vi "Create Test Library from Template.vi"() -> ()   [LabVIEW 2016]
doc: "This VI creates and adds the Drona test library template to the active project"
panel:
  out "error out":errorcluster
  in  "error in (no error)":errorcluster
  in  "Library Name":string="TestLibrary.lvlib"
  # "Creating Drona Test Library\nfrom Template......"
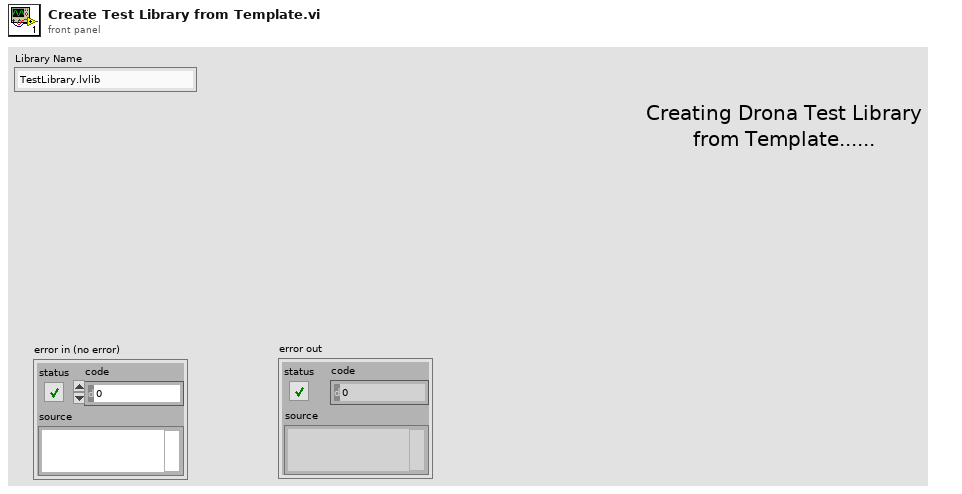
[diagram p1: front panel]
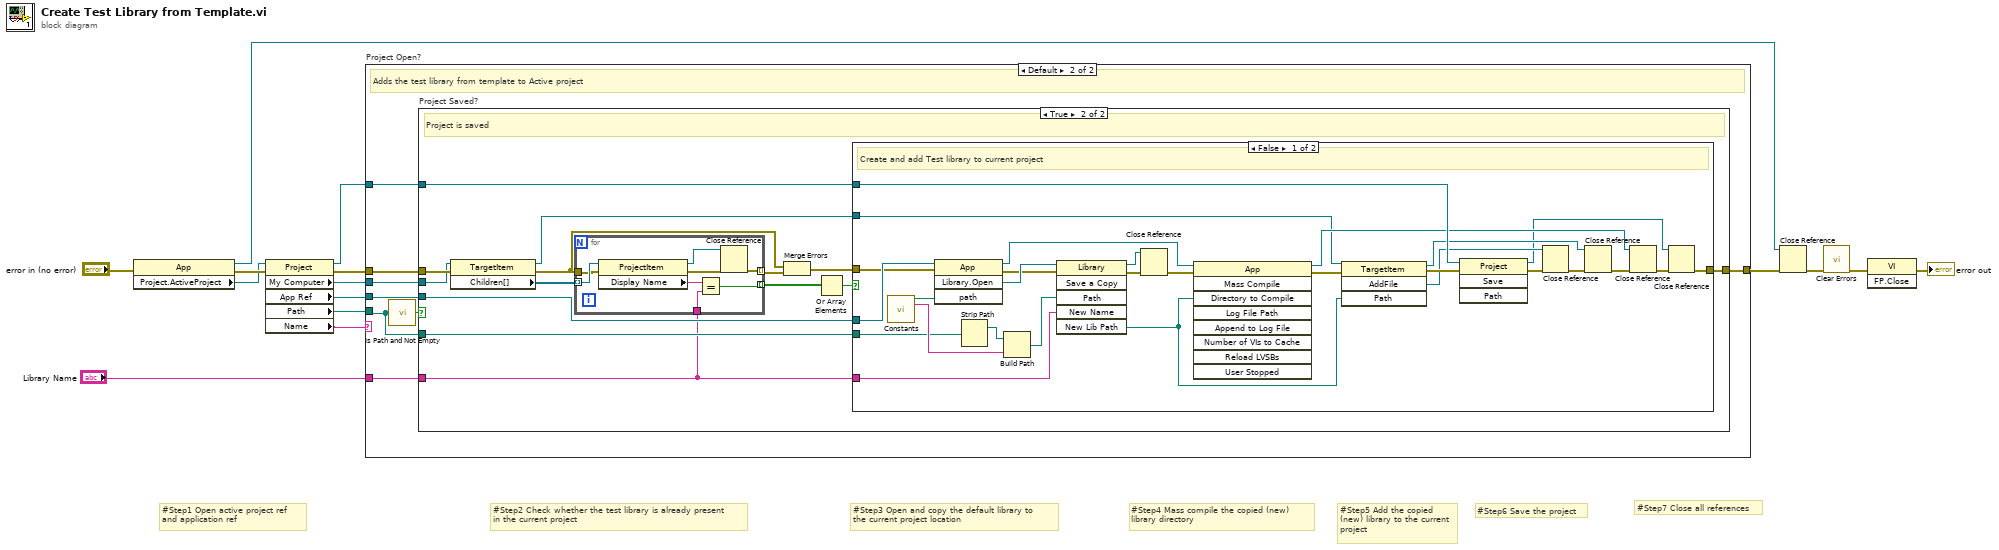
[diagram p0: block diagram]
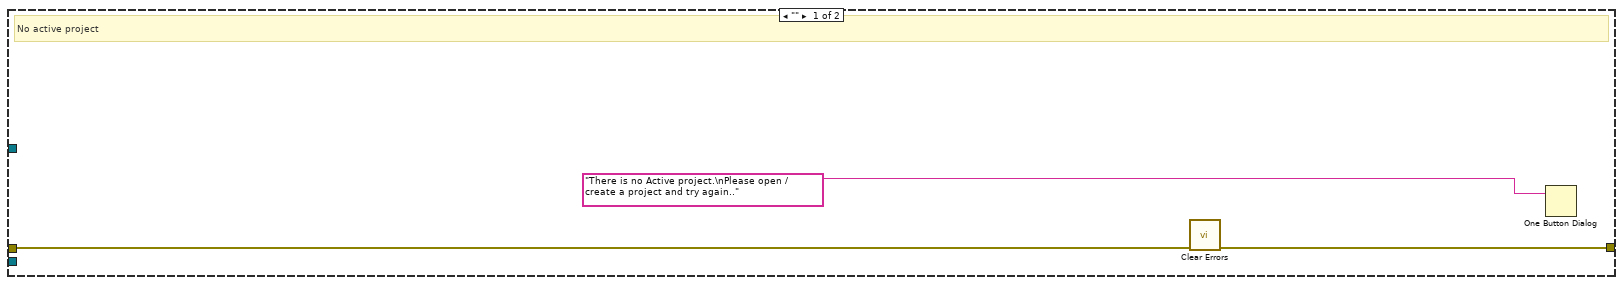
[diagram p2: hidden frame]
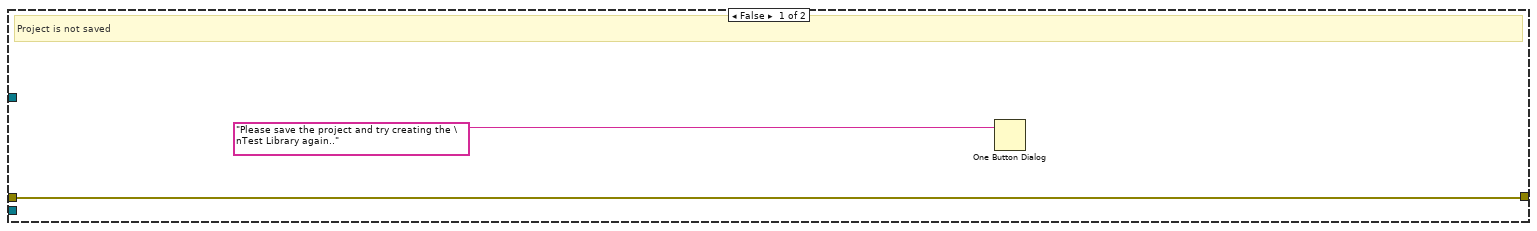
[diagram p3: hidden frame]
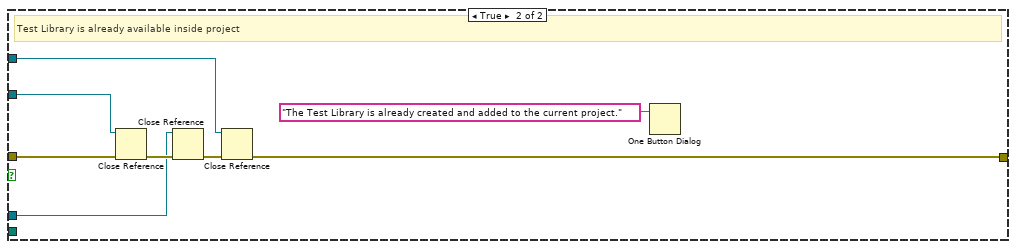
[diagram p4: hidden frame]
diagram:
  # "#Step7 Close all references"
  # "#Step6 Save the project"
  # "#Step5 Add the copied (new) library to the current project"
  # "#Step4 Mass compile the copied (new) \nlibrary directory"
  # "#Step3 Open and copy the default library to \nthe current project location"
  # "#Step2 Check whether the test library is already present\nin the current project"
  # "#Step1 Open active project ref \nand application ref"
  n1 = property class="App"(error in="error in (no error)") -> (reference out=w12:refnum<vi>, error out=w15:errorcluster, "Project.ActiveProject"=w11:refnum<vi>)  [unwired: 1 in]
  n2 = property class="Project"(reference=w11, error in=w15) -> (reference out=w2:refnum<vi>, error out=w14:errorcluster, "My Computer"=w3:refnum<vi>, "App Ref"=w13:refnum<vi>, "Path"=w10:path, "Name"=w9:string)
  n3 = case "Project Open?" shown="Default" w9 {
    tunnel: w3 -> [_ w21]
    tunnel: w14 -> [w18 w24]
    tunnel: w13 -> [_ w25]
    tunnel: [w17 w19] -> w1
    tunnel: w10 -> [_ w23]
    tunnel: "Library Name" -> [_ w22]
    tunnel: w2 -> [_ w20]
    frame "" {
      # "No active project"
      n4 = call <vilib>:"Clear Errors.vi"("error in (no error)"=w18) -> ("error out"=w17:errorcluster)  [unwired: 5 in, 1 out]
      n5 = One Button Dialog(message="There is no Active project.\nPlease open / create a project and try again..") -> ()  [unwired: 1 in, 1 out]
    }
    frame Default {
      # "Adds the test library from template to Active project"
      n6 = call <vilib>:"Is Path and Not Empty.vi"("path"=w23) -> ("Is Path and Not Empty?"=w26:bool)  [unwired: 4 in]
      n7 = case "Project Saved?" shown="True" w26 {
        tunnel: w25 -> [_ w42]
        tunnel: w24 -> [w28 w38]
        tunnel: w23 -> [_ w41]
        tunnel: w22 -> [_ w34]
        tunnel: w21 -> [_ w37]
        tunnel: w20 -> [_ w40]
        tunnel: [w28 w39] -> w19
        frame False {
          # "Project is not saved"
          n8 = One Button Dialog(message="Please save the project and try creating the \nTest Library again..") -> ()  [unwired: 1 in, 1 out]
        }
        frame True {
          # "Project is saved"
          n9 = property class="TargetItem"(reference=w37, error in=w38) -> (reference out=w36:refnum<vi>, error out=w31:errorcluster, "Children[]"=w35:refnum<vi>[])
          n10 = for {
            tunnel: w35 -> [w86] mode=indexing
            tunnel: w31 -> [w85]
            tunnel: w34 -> [w83]
            tunnel: [w82] -> w33 mode=indexing
            tunnel: [w79] -> w32 mode=indexing
            n11 = property class="ProjectItem"(reference=w86, error in=w85) -> (reference out=w81:refnum<vi>, error out=w80:errorcluster, "Display Name"=w84:string)
            n12 = Equal?(x=w84, y=w83) -> (x = y?=w82:bool)
            n13 = Close Reference(reference=w81, error in (no error)=w80) -> (error out=w79:errorcluster)
          }
          n14 = Merge Errors(w31, w32) -> (w30:errorcluster)
          n15 = Or Array Elements(Boolean array=w33) -> (logical OR=w29:bool)
          n16 = case shown="False" w29 {
            tunnel: w42 -> [w70 w76]
            tunnel: w41 -> [w64 _]
            tunnel: w40 -> [w55 w74]
            tunnel: [w46 w72] -> w39
            tunnel: w36 -> [w45 w78]
            tunnel: w34 -> [w44 _]
            tunnel: w30 -> [w43 w73]
            frame False {
              # "Create and add Test library to current project"
              n17 = call "Constants.vi"() -> ("VI path"=w69:path, "Tests folder name"=w65:string)  [unwired: 14 in]
              n18 = invoke class="App" method="Library.Open"(reference=w70, error in=w43, "path"=w69) -> (reference out=w60:refnum<vi>, error out=w67:errorcluster, "Open Library"=w68:refnum<vi>)  [unwired: 1 in, 1 out]
              n19 = Strip Path(path=w64) -> (stripped path=w66:path)  [unwired: 1 out]
              n20 = Build Path(base path=w66, name or relative path=w65) -> (appended path=w63:path)
              n21 = invoke class="Library" method="Save a Copy"(reference=w68, error in=w67, "Path"=w63, "New Name"=w44) -> (reference out=w61:refnum<vi>, error out=w62:errorcluster, "New Lib Path"=w57:path)  [unwired: 2 in, 3 out]
              n22 = Close Reference(reference=w61, error in (no error)=w62) -> (error out=w59:errorcluster)
              n23 = invoke class="App" method="Mass Compile"(reference=w60, error in=w59, "Directory to Compile"=w57) -> (reference out=w49:refnum<vi>, error out=w58:errorcluster)  [unwired: 6 in, 7 out]
              n24 = invoke class="TargetItem" method="AddFile"(reference=w45, error in=w58, "Path"=w57) -> (reference out=w51:refnum<vi>, error out=w56:errorcluster, "AddFile"=w52:refnum<vi>)  [unwired: 1 in, 1 out]
              n25 = invoke class="Project" method="Save"(reference=w55, error in=w56) -> (reference out=w47:refnum<vi>, error out=w54:errorcluster)  [unwired: 2 in, 2 out]
              n26 = Close Reference(reference=w52, error in (no error)=w54) -> (error out=w53:errorcluster)
              n27 = Close Reference(reference=w51, error in (no error)=w53) -> (error out=w50:errorcluster)
              n28 = Close Reference(reference=w49, error in (no error)=w50) -> (error out=w48:errorcluster)
              n29 = Close Reference(reference=w47, error in (no error)=w48) -> (error out=w46:errorcluster)
            }
            frame True {
              # "Test Library is already available inside project"
              n30 = Close Reference(reference=w78, error in (no error)=w73) -> (error out=w77:errorcluster)
              n31 = Close Reference(reference=w76, error in (no error)=w77) -> (error out=w75:errorcluster)
              n32 = Close Reference(reference=w74, error in (no error)=w75) -> (error out=w72:errorcluster)
              n33 = One Button Dialog(message="The Test Library is already created and added to the current project.") -> ()  [unwired: 1 in, 1 out]
            }
          }
        }
      }
    }
  }
  n34 = Close Reference(reference=w12, error in (no error)=w1) -> (error out=w6:errorcluster)
  n35 = call <vilib>:"Clear Errors.vi"("error in (no error)"=w6) -> ("error out"=w5:errorcluster)  [unwired: 5 in, 1 out]
  n36 = invoke class="VI" method="FP.Close"(error in=w5) -> (error out=→"error out":errorcluster)  [unwired: 2 in, 2 out]
